vi "Evaluate Invalid Fitness Solutions.vi"(8 "error in (no error)":errorcluster, 10 "OSSP_Problem.lvclass":refnum<class "OSSP_Problem.lvclass">, 11 "GA in":refnum<class "GA.lvclass">) -> (0 "error out":errorcluster, 2 "OSSP_Problem out":refnum<class "OSSP_Problem.lvclass">, 3 "GA out":refnum<class "GA.lvclass">)   [LabVIEW 2013, in "GA.lvclass"]
uses:
  GA.lvclass
  OSSP_Problem.lvclass
  GA.lvclass/GA.ctl
  GA_Operation_To_MachineJobTuple.vi
  Find Gaps On Particular Machine.vi
  GA_Check_Other_Machines.vi
  GA_Schedule_Job.vi
  GA_Find_Job_On_Other_Machines.vi
  GA_Increment_NumberofJobsOn Machine_ByOne.vi
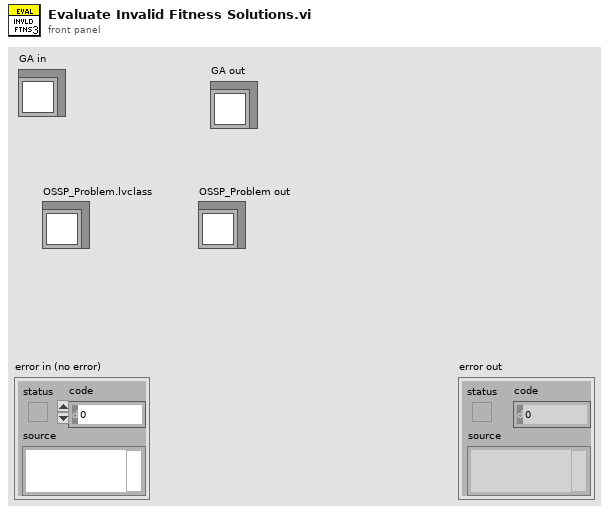
[diagram p1: front panel]
types:
  T1 = typedef "Solution.ctl" = cluster{"Schedule":u16[], "Fitness":u16, "Fitness Valid?":bool}
  T2 = typedef "GanntChart_Element.ctl" = cluster{"Operation Number":i32, "Job Number":i32, "Start Time":i32, "Procesing Time":u16, "End Time":i32}
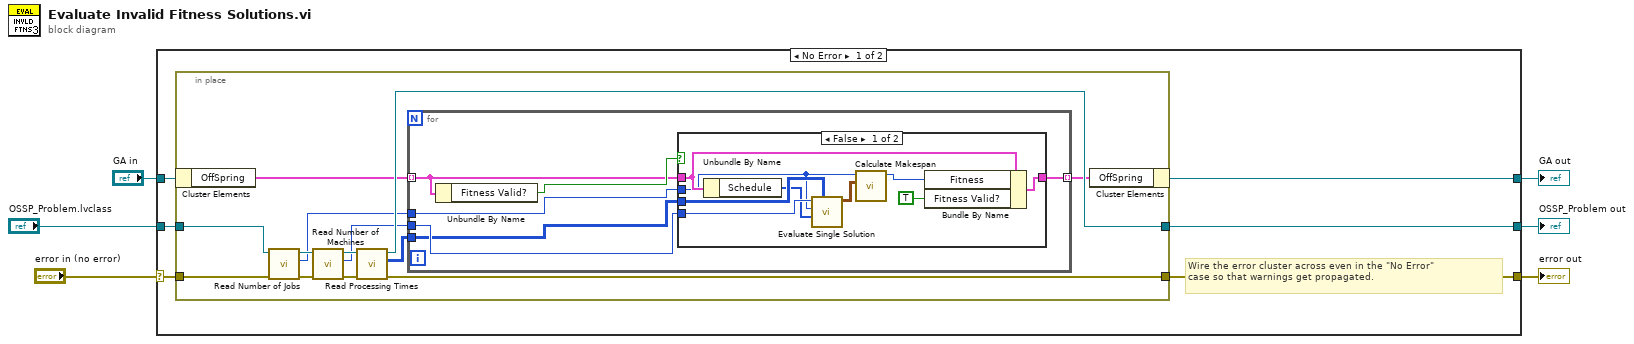
[diagram p0: block diagram]
diagram:
  n1 = case shown="No Error" "error in (no error)" {
    selector: "error in (no error)" -> [w10 w44]
    tunnel: [w9 w44] -> w5
    tunnel: [w7 w43] -> w3
    tunnel: "GA in" -> [w8 w43]
    tunnel: "OSSP_Problem.lvclass" -> [w12 w42]
    tunnel: [w11 w42] -> w1
    frame No Error {
      # "Wire the error cluster across even in the \"No Error\"\ncase so that warnings get propagated."
      n2 = in-place {
        in-place-border: w12 -> [w25]
        in-place-border: [w22] -> w11
        in-place-border: w10 -> [w16]
        in-place-border: [w15] -> w9
        n3 = in-place-cluster #1(w8) -> ("OffSpring"=w13:T1[])
        n4 = call-dynamic "Read Number of Jobs.vi"("error in (no error)"=w16, "OSSP_Problem in"=w25) -> ("error out"=w18:errorcluster, "Number of Jobs"=w21:i32, "OSSP_Problem out"=w24:refnum<class "OSSP_Problem.lvclass">)  [unwired: 7 in]
        n5 = call-dynamic "Read Number of Machines.vi"("error in (no error)"=w18, "OSSP_Problem in"=w24) -> ("error out"=w17:errorcluster, "Number of Machines"=w20:i32, "OSSP_Problem out"=w23:refnum<class "OSSP_Problem.lvclass">)  [unwired: 7 in]
        n6 = call-dynamic "Read Processing Times.vi"("error in (no error)"=w17, "OSSP_Problem in"=w23) -> ("error out"=w15:errorcluster, "Processing Times"=w19:u16[][], "OSSP_Problem out"=w22:refnum<class "OSSP_Problem.lvclass">)  [unwired: 7 in]
        n7 = for {
          tunnel: w13 -> [w30] mode=indexing
          tunnel: [w29] -> w14 mode=indexing
          tunnel: w21 -> [w28]
          tunnel: w20 -> [w27]
          tunnel: w19 -> [w26]
          n8 = Unbundle By Name(w30) -> ("Fitness Valid?"=w31:bool)
          n9 = case shown="False" w31 {
            tunnel: w30 -> [w39 w41]
            tunnel: [w40 w41] -> w29
            tunnel: w28 -> [w33 _]
            tunnel: w27 -> [w36 _]
            tunnel: w26 -> [w37 _]
            frame False {
              n10 = Unbundle By Name(w39) -> ("Schedule"=w35:u16[])
              n11 = call "Evaluate Single Solution.vi"("Processing Times (Rows Mach.Cols Jobs)"=w37, "Schedule"=w35, "Number of Jobs"=w33, "Number of Machines"=w36) -> ("Gannt Chart Out"=w34:T2[][])  [unwired: 7 in]
              n12 = call "Calculate Makespan.vi"("Gannt Chart Out"=w34, "Number of Jobs"=w33) -> ("Makespan"=w32:i32)  [unwired: 9 in]
              n13 = Bundle By Name(cluster=w39, "Fitness"=w32, "Fitness Valid?"=TRUE) -> (w40:T1)
            }
            frame True {
            }
          }
        }
        n14 = in-place-cluster #1("OffSpring"=w14) -> (w7:refnum<class "GA.lvclass">)
      }
    }
    frame Error {
    }
  }
  "error out" <- w5
  "GA out" <- w3
  "OSSP_Problem out" <- w1
